vi "建立模板.vi"(11 "输入MFCC":dbl[][](array[numeric])) -> ()   [LabVIEW 2018]
panel:
  out "Filename Out":path caption="文件名输出"
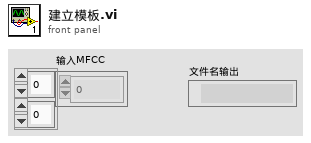
[diagram p1: front panel]
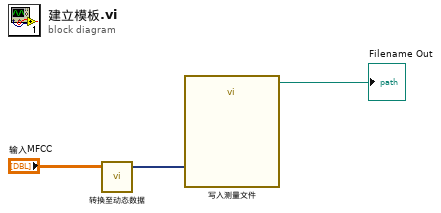
[diagram p0: block diagram]
diagram:
  n1 = call "转换至动态数据"("2D Array"="输入MFCC") -> ("Dynamic Data Type"=w3:dynamicdata)  [unwired: 3 in]
  n2 = call "写入测量文件"("Signals"=w3) -> ("Filename Out"=→"Filename Out":path)  [unwired: 16 in, 2 out]
